vi "Measurement Logic.vi"(8 "error in":errorcluster, 9 "Meas Config":T2={"Input Terminal Name"="Lorem ipsum dolor sit", "Counter Interface"="", "Active Edge"=1, "Pulses"=32, "Timeout (s)"=64, "FD Baudrate"=4294967264, "Baudrate"=4294967264, "FD ISO Mode"=enum."ISO", "IO Mode"=enum."CAN", "CAN Interface Name"="", "Termination CAN"=TRUE, "IDENTIFIER"=1, "PAYLOAD"=[3, 6], "TYPE"=0} {"TYPE" items=["CAN Data"=0, "CAN Remote"=1, "CAN Bus Error"=2, "CAN 2.0 Data"=8, "CAN FD Data"=16, "CAN FD+BRS Data"=24, "J1939 Data"=192, "Delay"=224, "Log Trigger"=225, "Start Trigger"=226]; "PAYLOAD" format="%x"; "IDENTIFIER" format="%x"; "Baudrate" format="%x"; "FD Baudrate" format="%x"; "Active Edge" items=["Rising"=10280, "Falling"=10171]}, 10 "measure call context in":refnum<class "Measure Call Context.lvclass">) -> (0 "error out":errorcluster, 1 "measurement results":T1, 2 "measure call context out":refnum<class "Measure Call Context.lvclass">)   [LabVIEW 2025, in "Workflow DO.lvclass"]
doc: "Contains the core logic for executing the measurement."
uses:
  Workflow DO.lvclass
  <vilib>/Plug-In SDKs/Measurements/Measure Call Context/Measure Call Context.lvclass
  Measurement Configuration.ctl
  Measurement Results.ctl
  <vilib>/DAQmx/read.llb/DAQmx Read (Counter U32 1Chan 1Samp).vi
  <vilib>/xnet/xnet.llb/XNET Read (Frame CAN).vi
  <vilib>/DAQmx/miscellaneous.llb/DAQmx Fill In Error Info.vi
  <extravilib>/ChannelInstances/Event Messenger-bool/Instantiate.vi
  Workflow DO.lvclass/Workflow DO.ctl
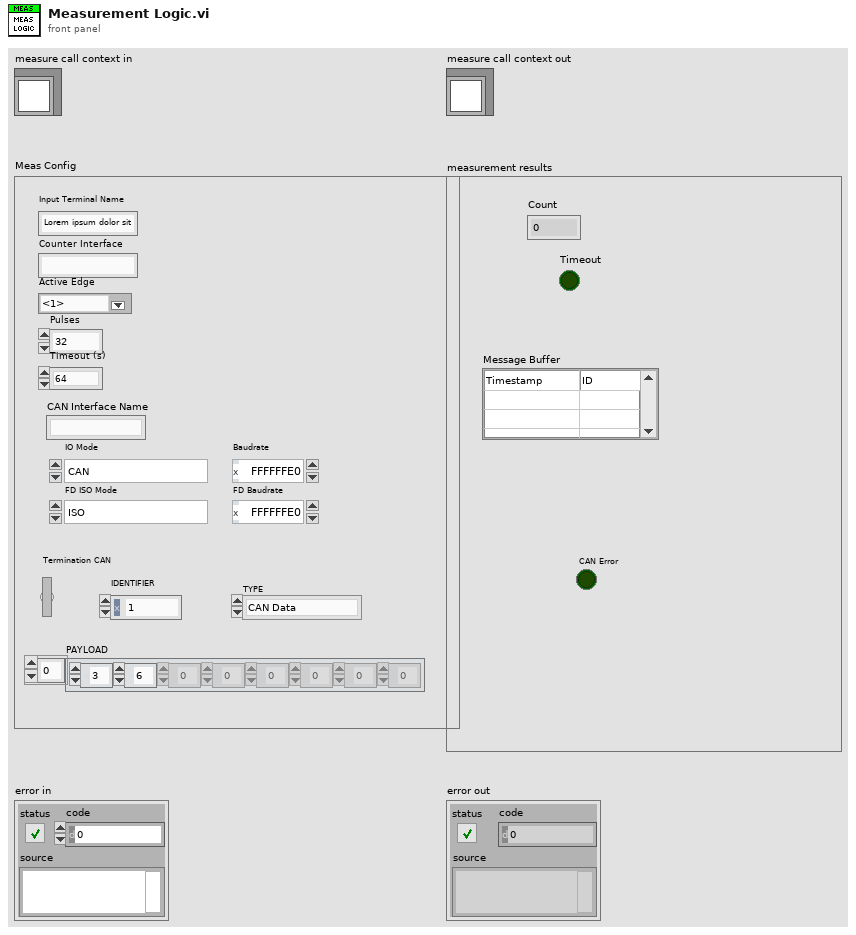
[diagram p1: front panel]
types:
  T1 = typedef "Workflow DO.lvclass/Measurement Results.ctl" = cluster{"Count":u32, "Timeout":bool, "Message Buffer":string[][], "CAN Error":bool}
  T2 = typedef "Workflow DO.lvclass/Measurement Configuration.ctl" = cluster{"Input Terminal Name":string, "Counter Interface":string, "Active Edge":i32, "Pulses":u32, "Timeout (s)":u32, "FD Baudrate":u32, "Baudrate":u32, "FD ISO Mode":enum32{"ISO", "Legacy ISO", "Non-ISO"}, "IO Mode":enum32{"CAN", "CAN FD", "CAN FD + BRS"}, "CAN Interface Name":string, "Termination CAN":bool, "IDENTIFIER":u32, "PAYLOAD":u32[], "TYPE":u32}
  T3 = typedef "XNET Frame CAN.ctl" = cluster{"timestamp":timestamp, "payload":u8[], "identifier":u32, "type":T4, "extended?":bool, "echo?":bool}
  T4 = typedef "XNET Frame Type CAN.ctl" = u8
  T5 = typedef "Event Messenger-bool.lvlib/))Channel.ctl" = refnum<queue>
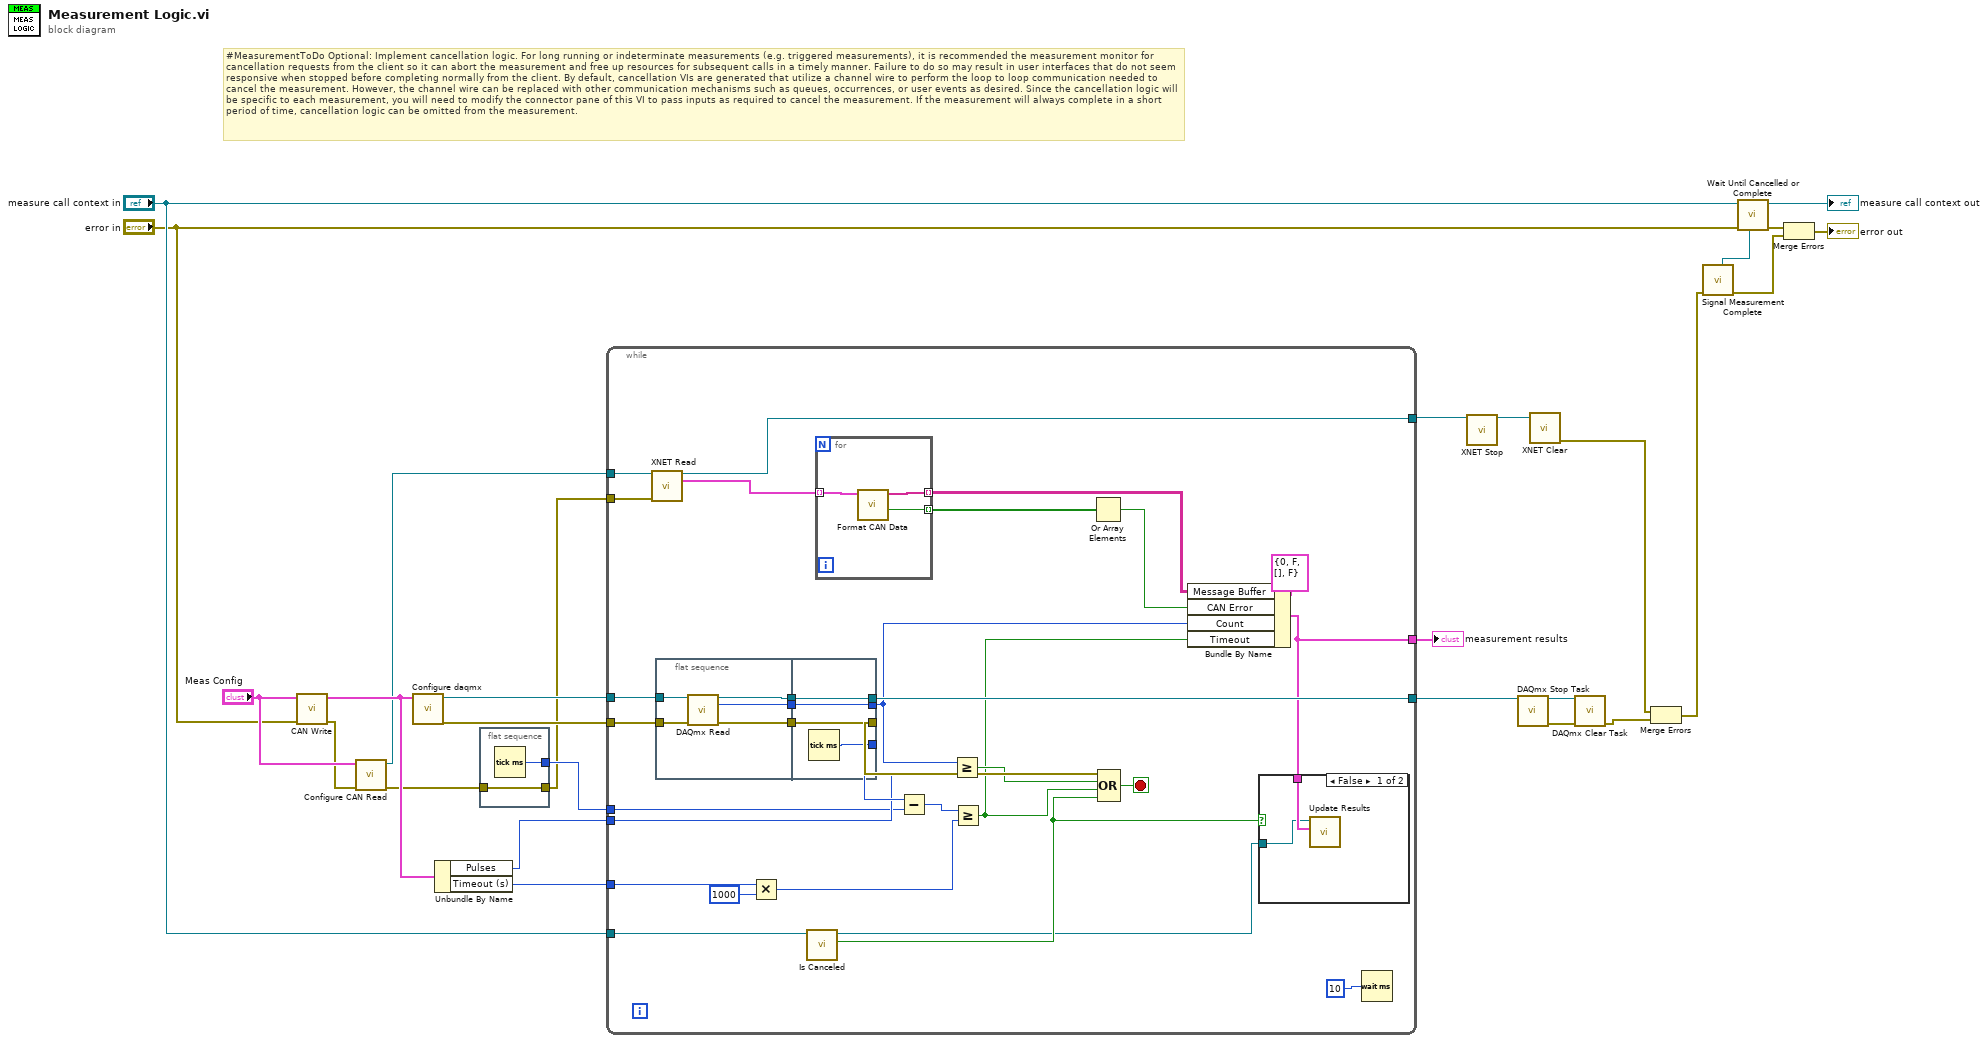
[diagram p0: block diagram]
diagram:
  # "#MeasurementToDo Optional: Implement cancellation logic. For long running or indeterminate measurements (e.g. triggered measurements), it is recommended the measurement monitor for cancellation requests from the client so it can abort the measurement and free up resources for subsequent calls in a timely manner. Failure to do so may result in user interfaces that do not seem responsive when stopped before completing normally from the client. By default, cancellation VIs are generated that utilize a channel wire to perform the loop to loop communication needed to cancel the measurement. However, the channel wire can be replaced with other communication mechanisms such as queues, occurrences, or user events as desired. Since the cancellation logic will be specific to each measurement, you will need to modify the connector pane of this VI to pass inputs as required to cancel the measurement. If the measurement will always complete in a short period of time, cancellation logic can be omitted from the measurement."
  n1 = call "CAN Write.vi"("error in"="error in", "Meas Config"="Meas Config") -> ("error out"=w9:errorcluster, "Meas Config"=w18:T2)  [unwired: 7 in, 1 out]
  n2 = call "Configure CAN Read.vi"("error in"=w9, "measurement configuration"="Meas Config") -> ("error out"=w4:errorcluster, "XNET Read"=w10:refnum<k21>)  [unwired: 8 in]
  n3 = call "Configure daqmx.vi"("measurement configuration"=w18) -> ("error out"=w7:errorcluster, "Task out"=w16:refnum<k21>)  [unwired: 9 in]
  n4 = Unbundle By Name(w18) -> ("Pulses"=w15:u32, "Timeout (s)"=w17:u32)
  n5 = flat-sequence {
    tunnel: [w29] -> w8
    tunnel: w4 -> [w28]
    tunnel: [w28] -> w3
    frame #0 {
      n6 = Tick Count (ms)() -> (millisecond timer value=w29:u32)
    }
  }
  n7 = while {
    tunnel: "measure call context in" -> [w57]
    tunnel: w16 -> [w43]
    tunnel: [w60] -> w20
    tunnel: w17 -> [w47]
    tunnel: w15 -> [w48]
    tunnel: w10 -> [w42]
    tunnel: [w41] -> w5
    tunnel: w8 -> [w40]
    tunnel: w7 -> [w39]
    tunnel: w3 -> [w38]
    tunnel: [w35] -> w2
    stop <- w58 stop-if-true
    n8 = call-poly <vilib>:"XNET Read.vi"("session in"=w42, "error in (no error)"=w38) -> ("session out"=w41:refnum<k21>, "data"=w33:T3[])  [unwired: 10 in, 2 out]
    n9 = flat-sequence {
      tunnel: [w68] -> w55
      tunnel: [w67] -> w54
      tunnel: [w66] -> w53
      tunnel: w43 -> [w65]
      tunnel: w39 -> [w64]
      tunnel: [w70] -> w56
      tunnel: [w71] -> w50
      tunnel: [w72] -> w60
      tunnel: w55 -> [w72]
      tunnel: w54 -> [w71]
      tunnel: w53 -> [w70]
      tunnel: [w69] -> w52
      frame #0 {
        n10 = call-poly <vilib>:"DAQmx Read.vi"("task/channels in"=w65, "error in"=w64) -> ("task out"=w68:refnum<k21>, "data"=w67:u32, "error out"=w66:errorcluster)  [unwired: 11 in]
      }
      frame #1 {
        n11 = Tick Count (ms)() -> (millisecond timer value=w69:u32)
      }
    }
    n12 = Multiply(x=w47, y=u32 1000) -> (x*y=w45:u32)
    n13 = call <vilib>:"Is Canceled.vi"("measure call context in"=w57) -> ("is canceled?"=w36:bool, "measure call context out"=w34:refnum<class "Measure Call Context.lvclass">)  [unwired: 8 in, 1 out]
    n14 = for {
      tunnel: w33 -> [w62] mode=indexing
      tunnel: [w63] -> w31 mode=indexing
      tunnel: [w61] -> w32 mode=indexing
      n15 = call "Format CAN Data.vi"("Frame"=w62) -> ("Error"=w61:bool, "Display"=w63:string[])  [unwired: 8 in, 1 out]
    }
    n16 = Subtract(x=w52, y=w40) -> (x-y=w51:u32)
    n17 = Greater Or Equal?(x=w50, y=w48) -> (x >= y?=w49:bool)
    n18 = Greater Or Equal?(x=w51, y=w45) -> (x >= y?=w46:bool)
    n19 = Or Array Elements(Boolean array=w32) -> (logical OR=w30:bool)
    n20 = Compound Arithmetic op=OR(w56, w49, w46, w36) -> (w58:bool)
    n21 = Bundle By Name(cluster=T1 {"Count"=0, "Timeout"=FALSE, "Message Buffer"=[], "CAN Error"=FALSE} ("measurement results"), "Message Buffer"=w31, "CAN Error"=w30, "Count"=w50, "Timeout"=w46) -> (w35:T1)
    n22 = case shown="False" w36 {
      tunnel: w35 -> [w74 _]
      tunnel: w34 -> [w73 _]
      frame False {
        n23 = call <vilib>:"Update Results.vi"("measurement results"=w74, "measure call context in"=w73) -> ()  [unwired: 8 in, 2 out]
      }
      frame True {
      }
    }
    n24 = Wait (ms)(milliseconds to wait=u32 10 ("Loop Time (ms)")) -> ()  [unwired: 1 out]
  }
  "measurement results" <- w2
  n25 = call <vilib>:"XNET Stop.vi"("session in"=w5) -> ("session out"=w6:refnum<k21>)  [unwired: 13 in, 1 out]
  n26 = call <vilib>:"DAQmx Stop Task.vi"("task/channels in"=w20) -> ("task out"=w21:refnum<k21>, "error out"=w22:errorcluster)  [unwired: 13 in]
  n27 = call <vilib>:"XNET Clear.vi"("session in"=w6) -> ("error out"=w1:errorcluster)  [unwired: 14 in]
  n28 = call <vilib>:"DAQmx Clear Task.vi"("task in"=w21, "error in"=w22) -> ("error out"=w19:errorcluster)  [unwired: 13 in]
  n29 = Merge Errors(w1, w19) -> (w11:errorcluster)
  n30 = call "Signal Measurement Complete.vi"("error in (no error)"=w11) -> ("error out"=w25:errorcluster, "done channel"=w26:T5)  [unwired: 9 in]
  n31 = call "Wait Until Cancelled or Complete.vi"("done channel"=w26, "error in (no error)"="error in", "measure call context in"="measure call context in") -> ("error out"=w24:errorcluster, "measure call context out"=→"measure call context out":refnum<class "Measure Call Context.lvclass">)  [unwired: 7 in]
  n32 = Merge Errors(w24, w25) -> (→"error out":errorcluster)
